vi "ZDataVIS_Retrieve_Engine.vi"(0 "File or Folder Path":path=path "C:/Users/voodoo/Desktop/IV_separat_Vsgsweep_2fields_Vbg-2.8V", 1 "attempt to fix filtered time?":bool, 2 "decimating factor":i32=1, 5 "offset":i32, 7 "length":i32, 9 "base processed path":path=path "C:/Users/voodoo/Desktop/IV_separat_Vsgsweep_2fields_Vbg-2.8V", 11 "Only Read 1st YAML":bool, 12 "Parse YAML Lockin Info":bool, 13 "decimate files (1 for no)":i32=1) -> (4 "generated files":path[](array[path]), 6 "Index, Wavenames":string[][](array[string]), 8 "clean names":string[](array[string]), 10 "all lockin AO":T1[](array[typedef]) {"AO f (Hz)" min=0.001 max=10000.0; "AO DC (V)" format="%.3p"; "AO Amp (V)" format="%.3p"}, 14 "wirings":string[][][](array[string]), 15 "ITX sizes (#chan and #samp)":i32[](array[numeric]))   [LabVIEW 2016]
uses:
  <userlib>/LevyLab/Lockin-Multichannel/Instrument.Lockin/Typedefs/AO-cluster.ctl
  <userlib>/LevyLab/Lockin-Multichannel/Instrument.Lockin/Typedefs/AO_Amp-array.ctl
  <userlib>/LevyLab/Lockin-Multichannel/Instrument.Lockin/Typedefs/AO_DC-array.ctl
  <userlib>/LevyLab/Lockin-Multichannel/Instrument.Lockin/Typedefs/AO_f-array.ctl
  <userlib>/LevyLab/Lockin-Multichannel/Instrument.Lockin/Typedefs/AO_phi-array.ctl
  <userlib>/LevyLab/Lockin-Multichannel/Instrument.Lockin/Typedefs/Function-array.ctl
  <userlib>/LevyLab/Lockin-Multichannel/Instrument.Lockin/Typedefs/Function-enum.ctl
  <vilib>/Analysis/NI_AALPro.lvlib
  <vilib>/Analysis/2dsp.llb/Decimate (single shot, DBL).vi
  <userlib>/LevyLab/Lockin-Multichannel/Instrument.Lockin/Instrument.Lockin.lvclass
panel:
  out "wiring":string[][](array[string])
  # "1"
  # "2"
  # "3"
  # "4"
  # "5"
  # "6"
  # "7"
  # "8"
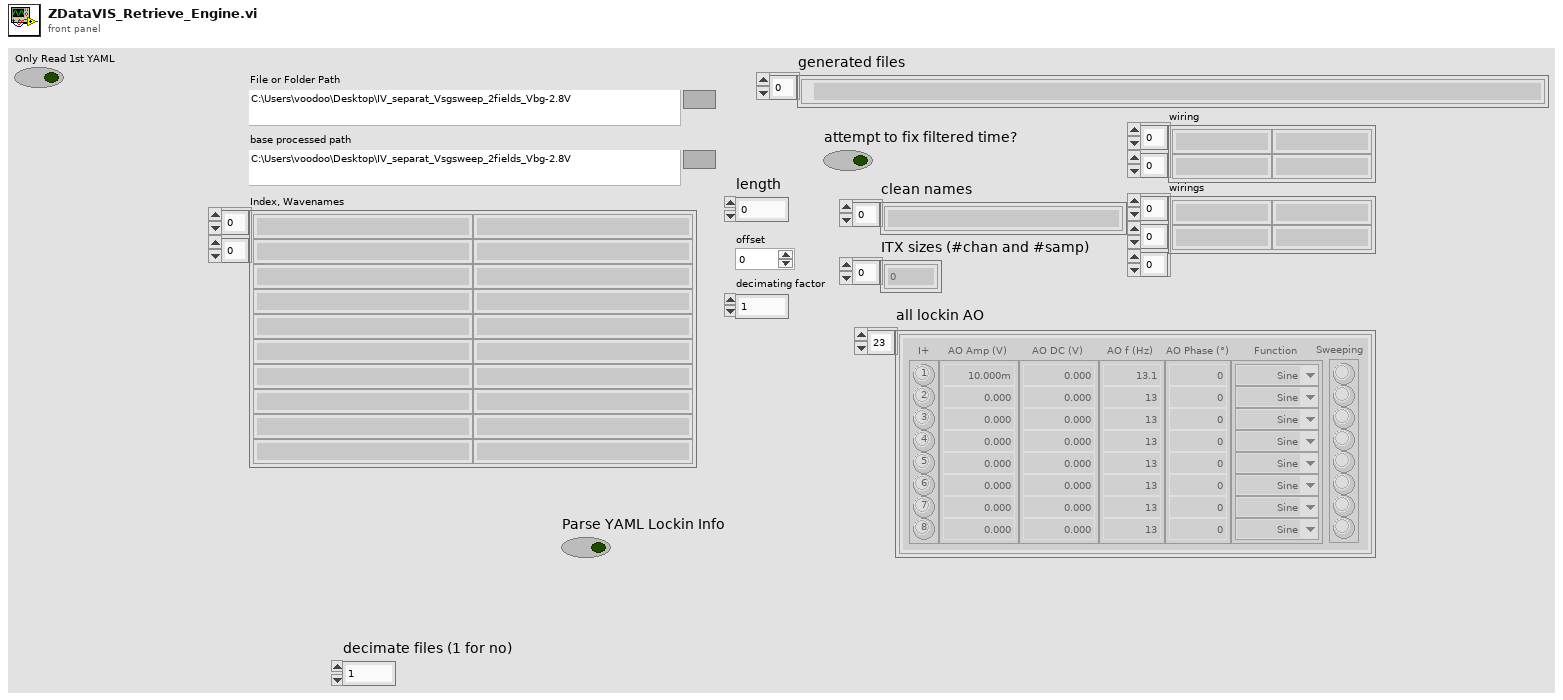
[diagram p1: front panel]
types:
  T1 = typedef "Instrument.Lockin.lvclass/AO-cluster.ctl" = cluster{"AO Amp (V)":T2, "AO DC (V)":T3, "AO f (Hz)":T4, "AO Phase (°)":T5, "Function":T6, "I+":bool[], "Sweeping":bool[]}
  T2 = typedef "Instrument.Lockin.lvclass/AO_Amp-array.ctl" = dbl[]
  T3 = typedef "Instrument.Lockin.lvclass/AO_DC-array.ctl" = dbl[]
  T4 = typedef "Instrument.Lockin.lvclass/AO_f-array.ctl" = dbl[]
  T5 = typedef "Instrument.Lockin.lvclass/AO_phi-array.ctl" = dbl[]
  T6 = typedef "Instrument.Lockin.lvclass/Function-array.ctl" = T7[]
  T7 = typedef "Instrument.Lockin.lvclass/Function-enum.ctl" = enum16{"Sine", "Triangle", "Square", "Sawtooth"}
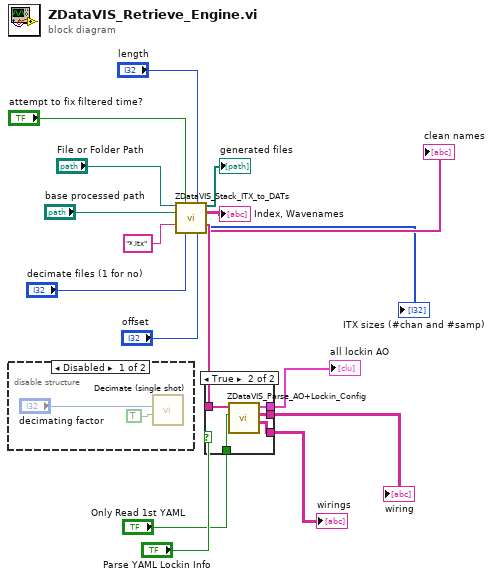
[diagram p0: block diagram]
diagram:
  n1 = disable-structure shown="Disabled" {
    frame Disabled {
      n2 = call-poly <vilib>:"Decimate (single shot).vi"("averaging"=TRUE, "decimating factor"="decimating factor") -> ()  [unwired: 8 in, 2 out]
    }
    frame Enabled {
    }
  }
  n3 = call "ZDataVIS_Stack_ITX_to_DATs.vi"("File or Folder Path"="File or Folder Path", "attempt to fix filtered time?"="attempt to fix filtered time?", "length"="length", "base processed path"="base processed path", "pattern"="*.itx", "decimate files (1 for no)"="decimate files (1 for no)", "offset"="offset") -> ("generated files"=→"generated files":path[], "Index, Wavenames"=→"Index, Wavenames":string[][], "\"notes \""=w13:string[], "ITX sizes (#itx, #chan, #samp)"=→"ITX sizes (#chan and #samp)":i32[], "clean names"=→"clean names":string[])  [unwired: 4 in]
  n4 = case shown="True" "Parse YAML Lockin Info" {
    tunnel: w13 -> [_ w24]
    tunnel: [_ w23] -> w12
    tunnel: [_ w22] -> w3
    tunnel: [_ w21] -> w2
    tunnel: "Only Read 1st YAML" -> [_ w20]
    frame False {
    }
    frame True {
      n5 = call "ZDataVIS_Parse_AO+Lockin_Config.vi"("Only Read 1st YAML"=w20, "\"notes \""=w24) -> ("wirings"=w21:string[][][], "wiring"=w22:string[][], "all lockin AO"=w23:T1[])  [unwired: 7 in]
    }
  }
  "all lockin AO" <- w12
  "wiring" <- w3
  "wirings" <- w2
